vi "Run.vi"(8 "error in (no error)":errorcluster, 11 "Data Plugin in":refnum<class "Data Plugin.lvclass">) -> (0 "error out":errorcluster, 3 "Data Plugin out":refnum<class "Data Plugin.lvclass">)   [LabVIEW 2017, in "Data Engine.lvlib" / "Data Plugin.lvclass"]
uses:
  Data Plugin.lvclass
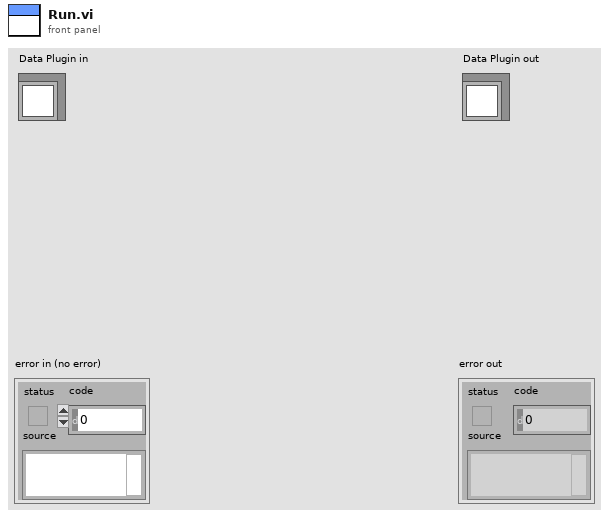
[diagram p1: front panel]
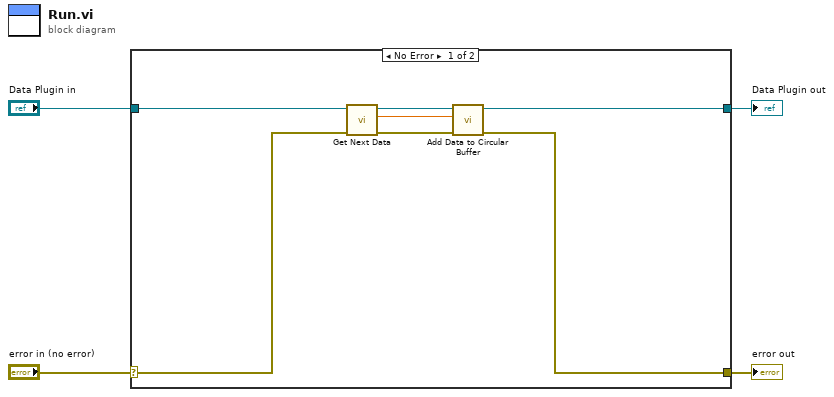
[diagram p0: block diagram]
diagram:
  n1 = case shown="No Error" "error in (no error)" {
    selector: "error in (no error)" -> [w6 w13]
    tunnel: [w5 w13] -> w3
    tunnel: [w8 w12] -> w1
    tunnel: "Data Plugin in" -> [w11 w12]
    frame No Error {
      n2 = call-dynamic "Get Next Data.vi"("error in (no error)"=w6, "Data Plugin in"=w11) -> ("error out"=w7:errorcluster, "Numeric"=w9:dbl, "Data Plugin out"=w10:refnum<class "Data Plugin.lvclass">)  [unwired: 7 in]
      n3 = call "Add Data to Circular Buffer.vi"("error in (no error)"=w7, "Data"=w9, "Data Plugin in"=w10) -> ("error out"=w5:errorcluster, "Data Plugin out"=w8:refnum<class "Data Plugin.lvclass">)  [unwired: 7 in]
    }
    frame Error {
    }
  }
  "error out" <- w3
  "Data Plugin out" <- w1
